vi "simon.vi"() -> ()   [LabVIEW 2024]
uses:
  state machine controller.ctl
  VI Communication.ctl
  HTTP_helpers/session.vi
  HTTP_helpers/user_name.vi
panel:
  in  "UI Controller":T1(tab)
  in  "Home page open leaderboard":bool caption="open leaderboard"
  in  "Home page login button":bool
  in  "Home page check rules":bool caption="Blank Button"
  in  "confirm login":bool
  in  "Login page go back":bool caption="Blank Button"
  in  "Login Password":string
  in  "User Name":string
  in  "Afterlogin Logout Button":bool
  out "user highest score achieved time":string
  out "user highest score":string
  out "Avatar":picture
  out "Afterlogin show user name":string
  in  "Afterlogin check leaderboard":bool caption="open leaderboard"
  in  "Afterlogin play":bool
  in  "AfterLogin home check rules":bool caption="Blank Button"
  in  "New Game":bool
  in  "Local Save":bool
  in  "Cloud Save":bool
  in  "How to start go back":bool caption="Blank Button"
  in  "Play Game":bool caption="Blank Button"
  in  "Difficulty":dbl(slide) scale=1.0..10.0
  in  "Difficulty go back":bool caption="Blank Button"
  in  "Game page EXIT":bool caption="Blank Button"
  out "Save Path":path
  out "Level":dbl
  out "Score":dbl
  in  "Pause Game Back to Home":bool
  # "Size 481 * 730"
  # "Simon Game"
  # "Login to play"
  # "Login or Register"
  # "User Name"
  # "Password"
  # "If you don't have an account yet, we will create one for you"
  # "Welcome"
  # "Simon Game"
  # "My highest score:"
  # "Achieved at:"
  # "How do you wanna start?"
  # "Your game will be automatically saved to server and \n./data/saves for local while playing"
  # "Difficulty?"
  # "Recommended"
  # "↓"
  # "Eazzzzzy"
  # "Hard"
  # "Your choice of difficulty will be counted in the score calculation"
  # "Session Finished"
  # "Score"
  # "Level"
  # "Save Path"
  # "Your game process is already saved on server"
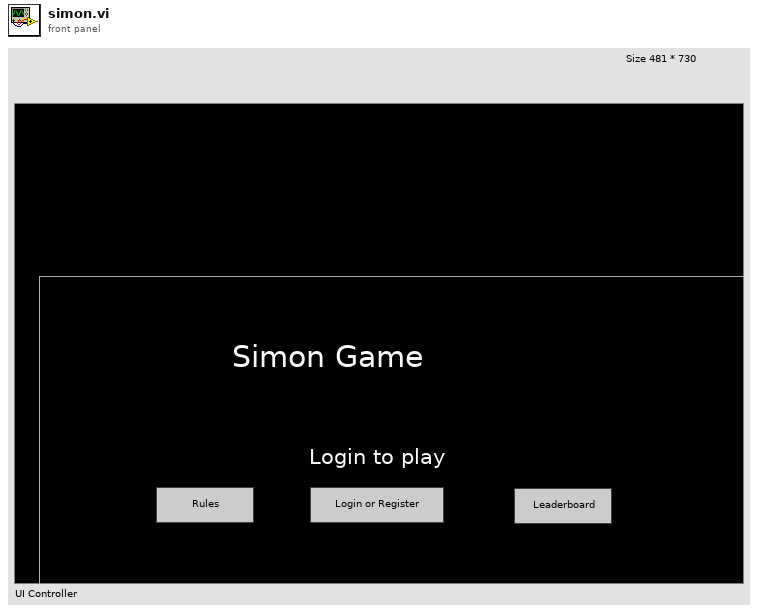
[diagram p1: front panel]
types:
  T1 = enum32{"Home Page", "Login Page", "AfterLogin Home", "How to Start", "New Game Difficulty", "Game Page", "Pause Game"}
  T2 = typedef "state machine controller.ctl" = cluster{"State Machine State":string, "Difficulty":dbl, "Login User Name":string, "Login User Passwd":string}
  T3 = enum32{"Home Page", "Login Page", "AfterLogin Home", "How to Start", "New Game Difficulty", "Game Page"}
  T4 = enum8{"Enabled", "Disabled", "Disabled and Grayed Out"}
  T5 = typedef "LVRectTypeDef.ctl" = cluster{"Left":i16, "Top":i16, "Right":i16, "Bottom":i16}
  T6 = typedef "imagedata.ctl" = cluster{"image type":i32, "image depth":i32, "image":u8[], "mask":u8[], "colors":u32[], "Rectangle":cluster{"left":i16, "top":i16, "right":i16, "bottom":i16}}
  T7 = typedef "VI Communication.ctl" = cluster{"Queue":refnum<queue>, "Path":path, "Score":dbl, "Level":dbl}
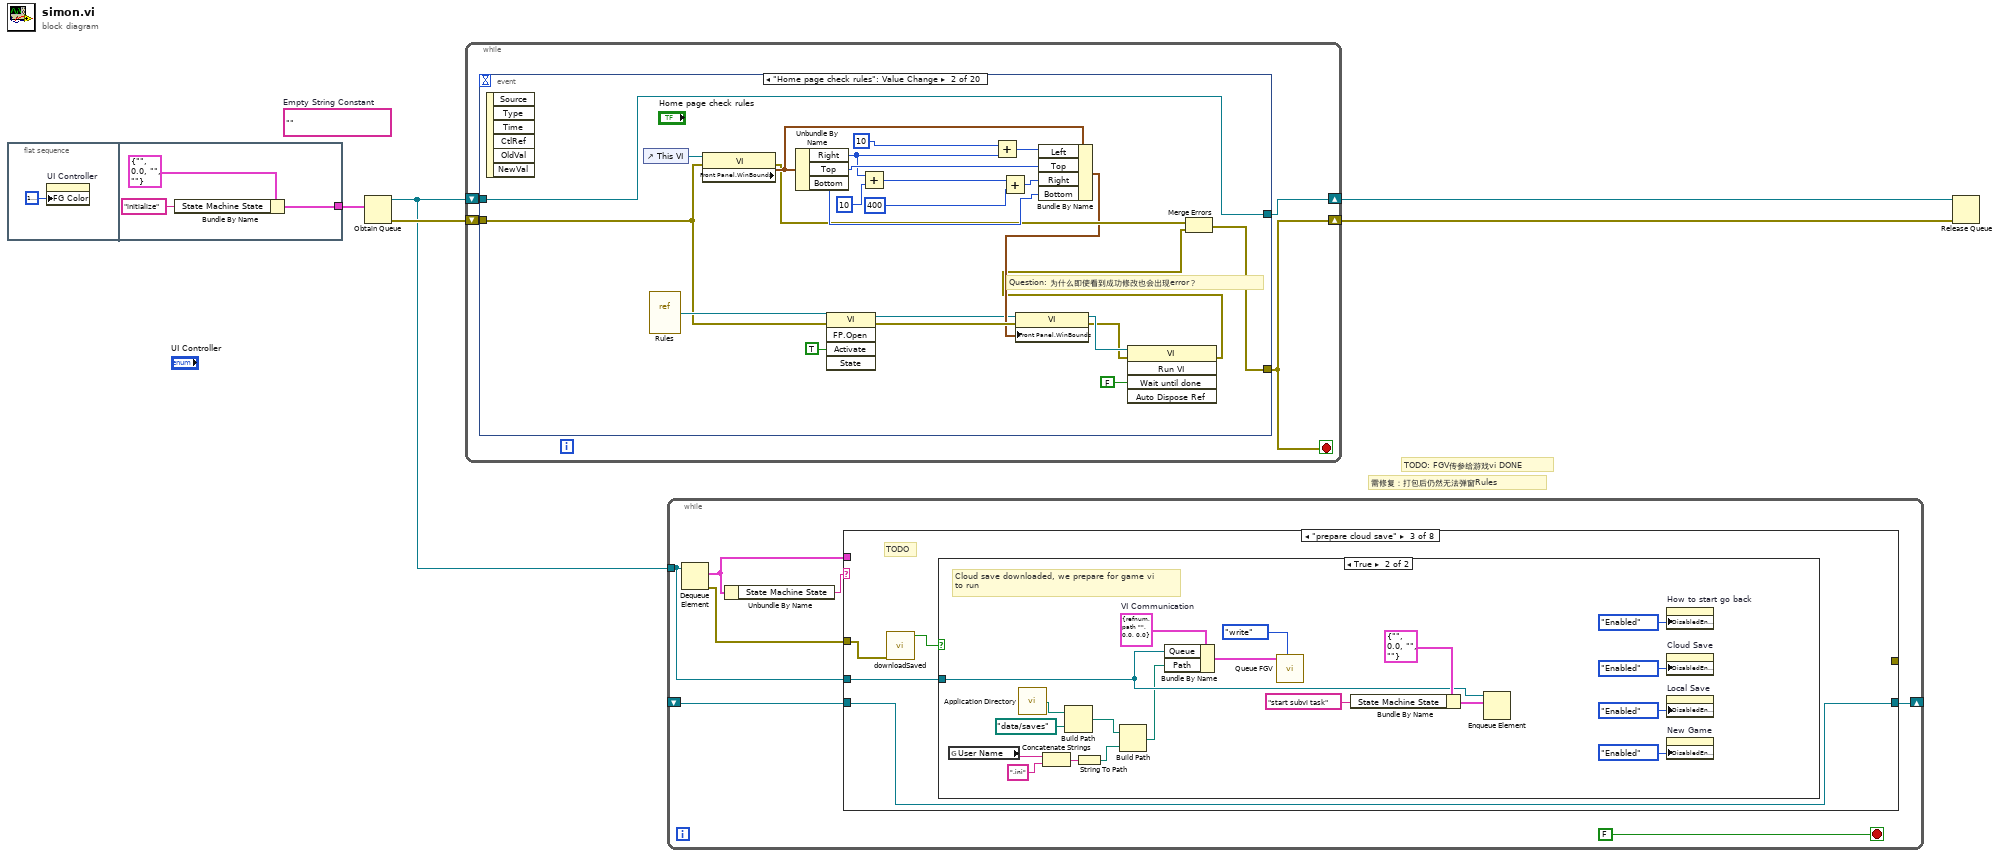
[diagram p0: block diagram]
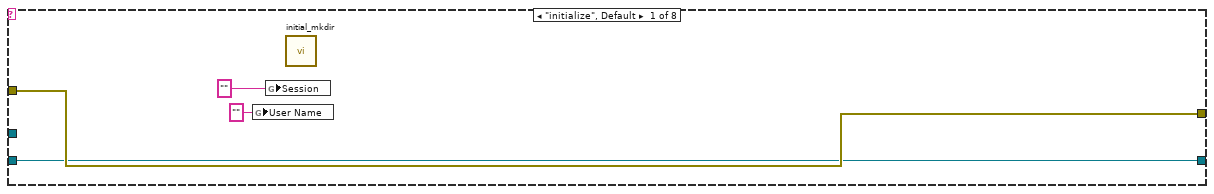
[diagram p2: hidden frame]
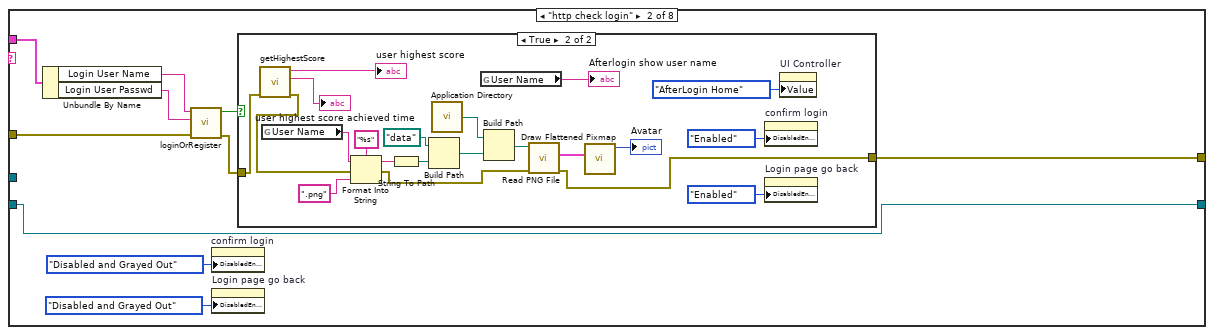
[diagram p3: hidden frame]
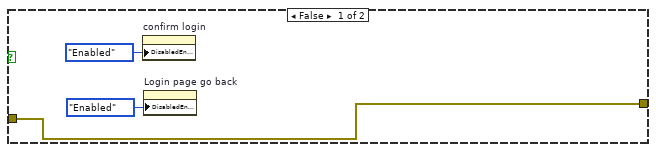
[diagram p4: hidden frame]
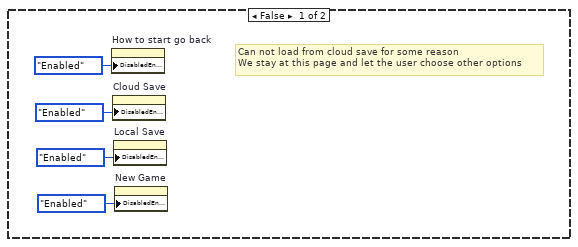
[diagram p5: hidden frame]
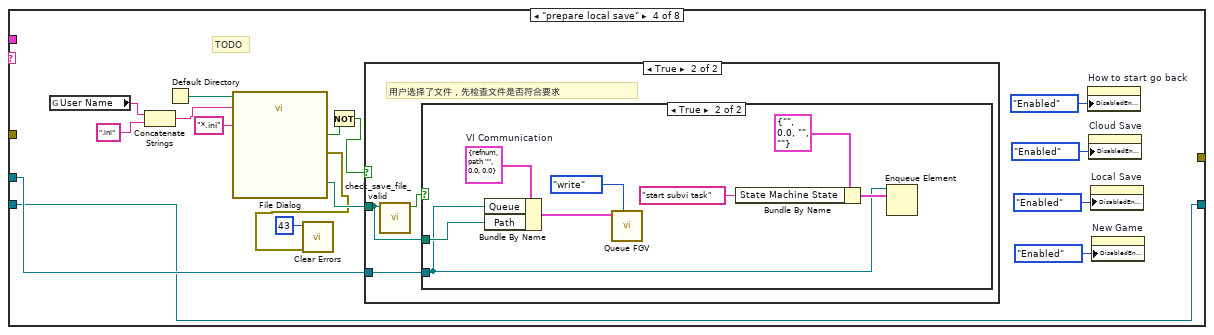
[diagram p6: hidden frame]
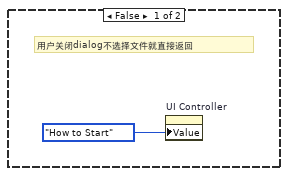
[diagram p7: hidden frame]
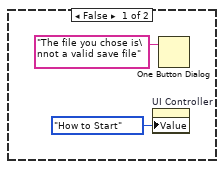
[diagram p8: hidden frame]
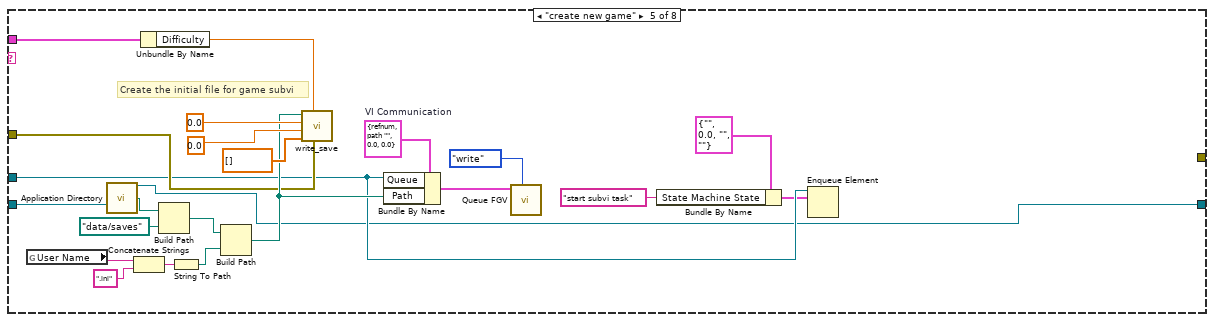
[diagram p9: hidden frame]
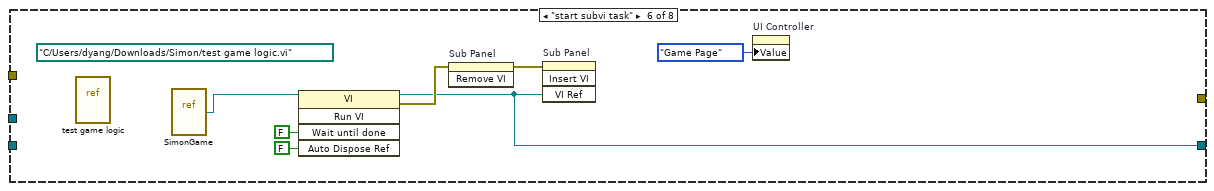
[diagram p10: hidden frame]
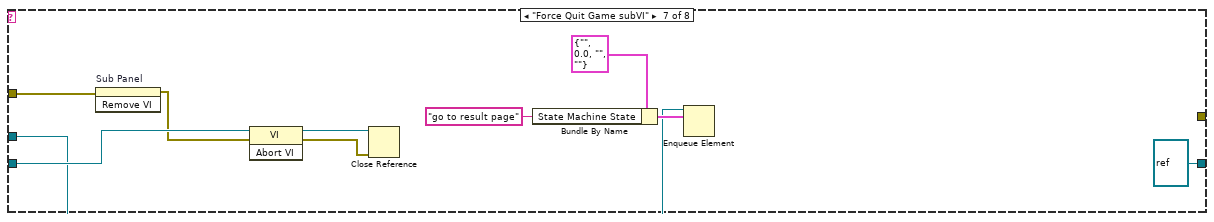
[diagram p11: hidden frame]
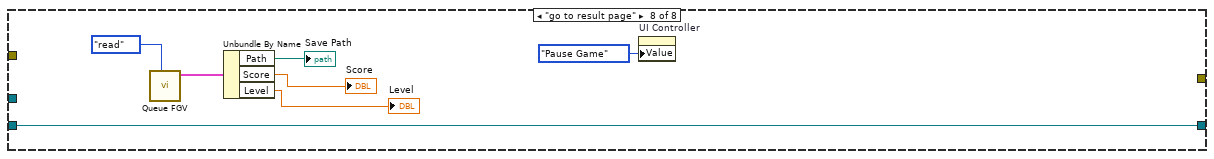
[diagram p12: hidden frame]
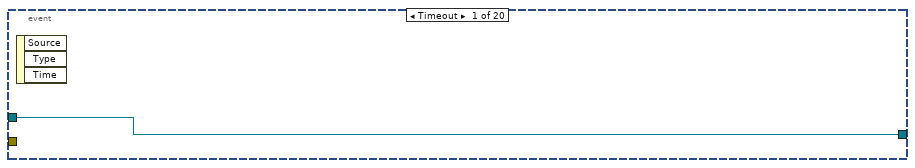
[diagram p13: hidden frame]
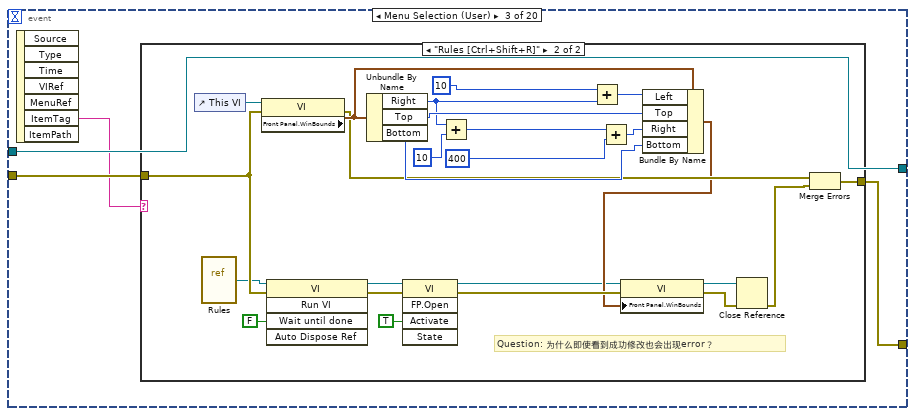
[diagram p14: hidden frame]
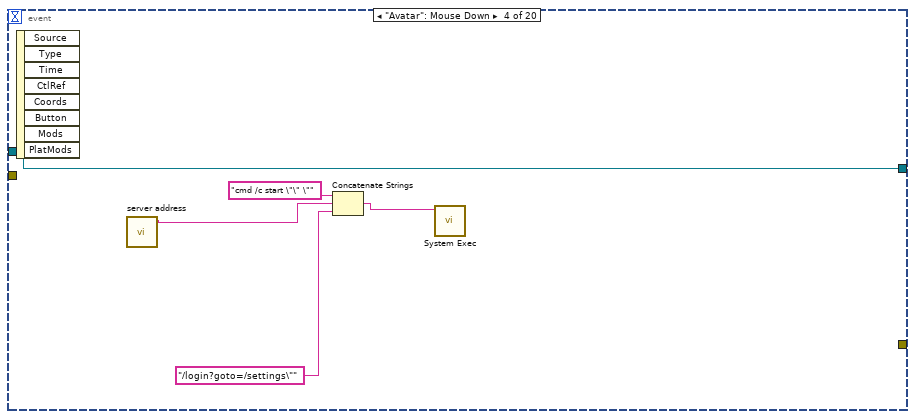
[diagram p16: hidden frame]
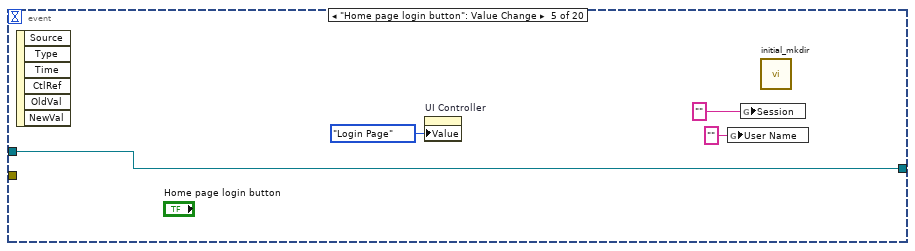
[diagram p17: hidden frame]
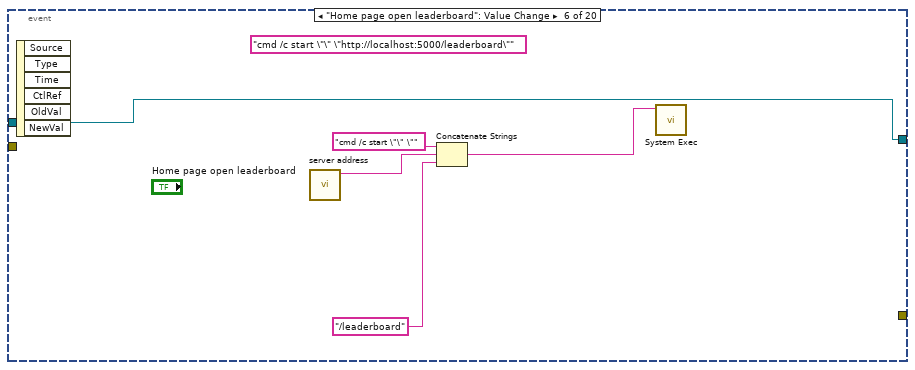
[diagram p18: hidden frame]
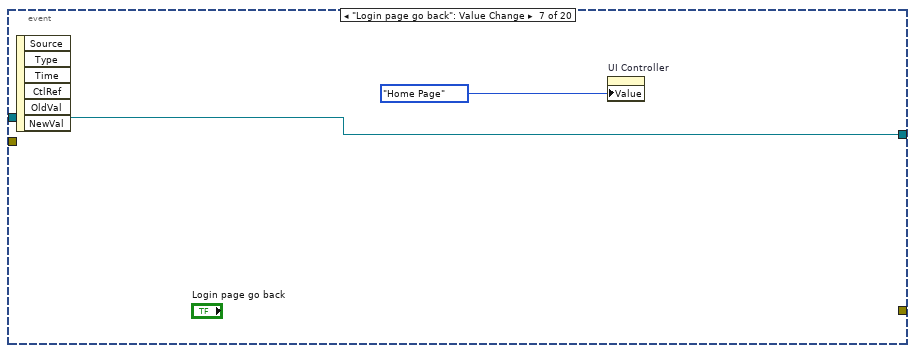
[diagram p19: hidden frame]
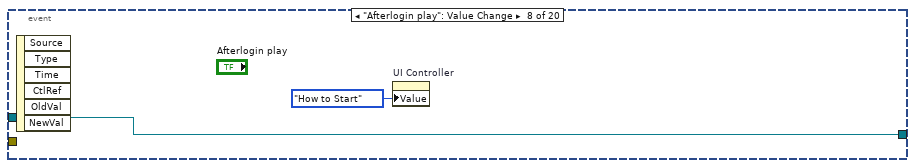
[diagram p20: hidden frame]
diagram:
  (unwired) ""  # Empty String Constant
  # "需修复：打包后仍然无法弹窗Rules"
  # "TODO: FGV传参给游戏vi DONE"
  n1 = flat-sequence {
    tunnel: [w7] -> w1
    frame #0 {
      n2 = property on="UI Controller" class="TabCtl (strict)"("FG Color"=u32 16777222 ("Colors:BG Color")) -> ()  [unwired: 2 in, 2 out]
    }
    frame #1 {
      n3 = Bundle By Name(cluster=T2 {"State Machine State"="", "Difficulty"=0.0, "Login User Name"="", "Login User Passwd"=""} ("Cluster"), "State Machine State"="initialize") -> (w7:T2)
    }
  }
  n4 = Obtain Queue(element data type=w1) -> (queue out=w2:refnum<queue>, error out=w5:errorcluster)  [unwired: 4 in, 1 out]
  n5 = while {
    shift-right: [w12] -> w4
    shift-left: w5 -> [w13]
    shift-right: [w11] -> w3
    shift-left: w2 -> [w10]
    stop <- w12 stop-if-true
    n6 = event shown="[1] \"Home page check rules\": Value Change" {
      selector: _ -> [_ _ _ _ _ _ _ _ _ _ _ _ _ _ _ _ _ _ _ _]
      dyn-events: _ -> [_ _ _ _ _ _ _ _ _ _ _ _ _ _ _ _ _ _ _ _]
      timeout: _ -> [_ _ _ _ _ _ _ _ _ _ _ _ _ _ _ _ _ _ _ _]
      tunnel: w13 -> [_ w18 w41 _ _ _ _ _ _ _ _ _ _ _ _ _ _ w134 _ _]
      tunnel: w10 -> [w14 w26 w42 w73 w76 w78 w83 w86 w88 w97 w106 w108 w110 w112 w118 w125 w127 w133 w161 w166]
      tunnel: [_ w25 w40 _ _ _ _ _ _ _ _ _ _ _ _ _ _ w138 _ _] -> w12
      tunnel: [w14 w26 w42 w73 w76 w78 w83 w86 w88 w96 w105 w108 w110 w113 w117 w125 w126 w133 w161 w166] -> w11
      event Timeout {
        n7 = event-data() -> ()  [unwired: 1 in, 3 out]
      }
      event "Home page check rules": Value Change {
        # "Question: 为什么即使看到成功修改也会出现error？"
        n8 = event-data() -> ()  [unwired: 1 in, 6 out]
        n9 = control-ref of="This VI"() -> (w38:refnum<vi>)
        n10 = vi-ref "Rules.vi"() -> (w19:refnum<vi>)
        n11 = property class="VI"(reference=w38, error in=w18) -> (error out=w27:errorcluster, "Front Panel.WinBounds"=w36:T5)  [unwired: 1 out]
        n12 = Unbundle By Name(w36) -> ("Right"=w33:i16, "Top"=w34:i16, "Bottom"=w28:i16)
        n13 = invoke class="VI" method="FP.Open"(reference=w19, error in=w18, "Activate"=TRUE ("Activate?")) -> (reference out=w20:refnum<vi>, error out=w22:errorcluster)  [unwired: 2 in, 3 out]
        n14 = Add(x=w33, y=i16 10) -> (x+y=w31:i16)
        n15 = Add(x=i16 10, y=w33) -> (x+y=w35:i16)
        n16 = Add(x=w31, y=i16 400) -> (x+y=w29:i16)
        n17 = Bundle By Name(cluster=w36, "Left"=w35, "Top"=w34, "Right"=w29, "Bottom"=w28) -> (w21:T5)
        n18 = property class="VI"(reference=w20, error in=w22, "Front Panel.WinBounds"=w21) -> (reference out=w17:refnum<vi>, error out=w16:errorcluster)
        n19 = invoke class="VI" method="Run VI"(reference=w17, error in=w16, "Wait until done"=FALSE ("Wait Until Done")) -> (error out=w15:errorcluster)  [unwired: 2 in, 4 out]
        n20 = Merge Errors(w27, w15) -> (w25:errorcluster)
      }
      event Menu Selection (User) {
        n21 = event-data() -> ("ItemTag"=w39:string)  [unwired: 1 in, 6 out]
        n22 = case shown="\"Rules [Ctrl+Shift+R]\"" w39 {
          tunnel: w41 -> [w43 w56]
          tunnel: [w43 w55] -> w40
          frame Default {
          }
          frame "Rules [Ctrl+Shift+R]" {
            # "Question: 为什么即使看到成功修改也会出现error？"
            n23 = control-ref of="This VI"() -> (w68:refnum<vi>)
            n24 = vi-ref "Rules.vi"() -> (w47:refnum<vi>)
            n25 = property class="VI"(reference=w68, error in=w56) -> (error out=w57:errorcluster, "Front Panel.WinBounds"=w66:T5)  [unwired: 1 out]
            n26 = invoke class="VI" method="Run VI"(reference=w47, error in=w56, "Wait until done"=FALSE ("Wait Until Done")) -> (reference out=w52:refnum<vi>, error out=w50:errorcluster)  [unwired: 2 in, 3 out]
            n27 = Unbundle By Name(w66) -> ("Right"=w63:i16, "Top"=w64:i16, "Bottom"=w58:i16)
            n28 = invoke class="VI" method="FP.Open"(reference=w52, error in=w50, "Activate"=TRUE ("Activate?")) -> (reference out=w44:refnum<vi>, error out=w46:errorcluster)  [unwired: 2 in, 3 out]
            n29 = Add(x=w63, y=i16 10) -> (x+y=w61:i16)
            n30 = Add(x=i16 10, y=w63) -> (x+y=w65:i16)
            n31 = Add(x=w61, y=i16 400) -> (x+y=w59:i16)
            n32 = Bundle By Name(cluster=w66, "Left"=w65, "Top"=w64, "Right"=w59, "Bottom"=w58) -> (w45:T5)
            n33 = property class="VI"(reference=w44, error in=w46, "Front Panel.WinBounds"=w45) -> (reference out=w49:refnum<vi>, error out=w48:errorcluster)
            n34 = Close Reference(reference=w49, error in (no error)=w48) -> (error out=w54:errorcluster)
            n35 = Merge Errors(w57, w54) -> (w55:errorcluster)
          }
        }
      }
      event "Avatar": Mouse Down {
        n36 = event-data() -> ()  [unwired: 1 in, 8 out]
        n37 = call "server address.vi"() -> ("Server Address"=w70:string)  [unwired: 11 in]
        n38 = Concatenate Strings("cmd /c start \"\" \"" ("string"), w70, "/login?goto=/settings\"" ("string")) -> (w69:string)
        n39 = call <vilib>:"System Exec.vi"("command line"=w69) -> ()  [unwired: 7 in, 4 out]
      }
      event "Home page login button": Value Change {
        n40 = event-data() -> ()  [unwired: 1 in, 6 out]
        n41 = property on="UI Controller" class="TabCtl (strict)"("Value"=T3."Login Page" ("UI Controller")) -> ()  [unwired: 2 in, 2 out]
        n42 = global write "user_name.vi" "User Name"("" ("User Name")) -> ()
        n43 = global write "session.vi" "Session"("" ("Session")) -> ()
        n44 = call "initial_mkdir.vi"() -> ()  [unwired: 11 in, 1 out]
      }
      event "Home page open leaderboard": Value Change {
        (unwired) "cmd /c start \"\" \"http://localhost:5000/leaderboard\"" ("command line")
        n45 = event-data() -> ()  [unwired: 1 in, 6 out]
        n46 = call "server address.vi"() -> ("Server Address"=w81:string)  [unwired: 11 in]
        n47 = Concatenate Strings("cmd /c start \"\" \"" ("string"), w81, "/leaderboard" ("string")) -> (w79:string)
        n48 = call <vilib>:"System Exec.vi"("command line"=w79) -> ()  [unwired: 7 in, 4 out]
      }
      event "Login page go back": Value Change {
        n49 = event-data() -> ()  [unwired: 1 in, 6 out]
        n50 = property on="UI Controller" class="TabCtl (strict)"("Value"=T3."Home Page" ("UI Controller")) -> ()  [unwired: 2 in, 2 out]
      }
      event "Afterlogin play": Value Change {
        n51 = event-data() -> ()  [unwired: 1 in, 6 out]
        n52 = property on="UI Controller" class="TabCtl (strict)"("Value"=T3."How to Start" ("UI Controller")) -> ()  [unwired: 2 in, 2 out]
      }
      event "How to start go back": Value Change {
        n53 = event-data() -> ()  [unwired: 1 in, 6 out]
        n54 = property on="UI Controller" class="TabCtl (strict)"("Value"=T3."AfterLogin Home" ("UI Controller")) -> ()  [unwired: 2 in, 2 out]
      }
      event "Cloud Save": Value Change {
        # "Check & Load Cloud Save from server"
        n55 = event-data() -> ()  [unwired: 1 in, 6 out]
        n56 = property on="Cloud Save" class="Bool"("DisabledEnum"=T4."Disabled and Grayed Out" ("Disabled")) -> ()  [unwired: 2 in, 2 out]
        n57 = property on="Local Save" class="Bool"("DisabledEnum"=T4."Disabled and Grayed Out" ("Disabled")) -> ()  [unwired: 2 in, 2 out]
        n58 = property on="How to start go back" class="Bool"("DisabledEnum"=T4."Disabled and Grayed Out" ("Disabled")) -> ()  [unwired: 2 in, 2 out]
        n59 = Bundle By Name(cluster=T2 {"State Machine State"="", "Difficulty"=0.0, "Login User Name"="", "Login User Passwd"=""} ("Cluster"), "State Machine State"="prepare cloud save") -> (w93:T2)
        n60 = Enqueue Element(queue=w97, element=w93) -> (queue out=w96:refnum<queue>)  [unwired: 2 in, 2 out]
        n61 = property on="New Game" class="Bool"("DisabledEnum"=T4."Disabled and Grayed Out" ("Disabled")) -> ()  [unwired: 2 in, 2 out]
      }
      event "Local Save": Value Change {
        n62 = event-data() -> ()  [unwired: 1 in, 6 out]
        n63 = property on="How to start go back" class="Bool"("DisabledEnum"=T4."Disabled and Grayed Out" ("Disabled")) -> ()  [unwired: 2 in, 2 out]
        n64 = property on="Cloud Save" class="Bool"("DisabledEnum"=T4."Disabled and Grayed Out" ("Disabled")) -> ()  [unwired: 2 in, 2 out]
        n65 = property on="Local Save" class="Bool"("DisabledEnum"=T4."Disabled and Grayed Out" ("Disabled")) -> ()  [unwired: 2 in, 2 out]
        n66 = property on="New Game" class="Bool"("DisabledEnum"=T4."Disabled and Grayed Out" ("Disabled")) -> ()  [unwired: 2 in, 2 out]
        n67 = Bundle By Name(cluster=T2 {"State Machine State"="", "Difficulty"=0.0, "Login User Name"="", "Login User Passwd"=""} ("Cluster"), "State Machine State"="prepare local save") -> (w102:T2)
        n68 = Enqueue Element(queue=w106, element=w102) -> (queue out=w105:refnum<queue>)  [unwired: 2 in, 2 out]
      }
      event "New Game": Value Change {
        n69 = event-data() -> ()  [unwired: 1 in, 6 out]
        n70 = property on="UI Controller" class="TabCtl (strict)"("Value"=T3."New Game Difficulty" ("UI Controller")) -> ()  [unwired: 2 in, 2 out]
      }
      event "Difficulty go back": Value Change {
        n71 = event-data() -> ()  [unwired: 1 in, 6 out]
        n72 = property on="UI Controller" class="TabCtl (strict)"("Value"=T3."How to Start" ("UI Controller")) -> ()  [unwired: 2 in, 2 out]
      }
      event "Play Game": Value Change {
        n73 = event-data() -> ()  [unwired: 1 in, 6 out]
        n74 = Bundle By Name(cluster=T2 {"State Machine State"="", "Difficulty"=0.0, "Login User Name"="", "Login User Passwd"=""} ("Cluster"), "State Machine State"="create new game", "Difficulty"="Difficulty") -> (w111:T2)
        n75 = Enqueue Element(queue=w112, element=w111) -> (queue out=w113:refnum<queue>)  [unwired: 2 in, 2 out]
      }
      event "Game page EXIT": Value Change {
        n76 = event-data() -> ()  [unwired: 1 in, 6 out]
        n77 = Bundle By Name(cluster=T2 {"State Machine State"="", "Difficulty"=0.0, "Login User Name"="", "Login User Passwd"=""} ("Cluster"), "State Machine State"="Force Quit Game subVI") -> (w119:T2)
        n78 = Enqueue Element(queue=w118, element=w119) -> (queue out=w117:refnum<queue>)  [unwired: 2 in, 2 out]
      }
      event "Pause Game Back to Home": Value Change {
        n79 = event-data() -> ()  [unwired: 1 in, 6 out]
        n80 = call "getHighestScore.vi"() -> ("Highest Score Achineved Time"=w122:string, "Highest Score"=w123:string)  [unwired: 9 in, 1 out]
        n81 = property on="user highest score" class="Str"("Value"=w123) -> ()  [unwired: 2 in, 2 out]
        n82 = property on="user highest score achieved time" class="Str"("Value"=w122) -> ()  [unwired: 2 in, 2 out]
        n83 = property on="UI Controller" class="TabCtl (strict)"("Value"=T1."AfterLogin Home" ("UI Controller")) -> ()  [unwired: 2 in, 2 out]
      }
      event "confirm login": Value Change {
        n84 = event-data() -> ()  [unwired: 1 in, 6 out]
        n85 = Bundle By Name(cluster=T2 {"State Machine State"="", "Difficulty"=0.0, "Login User Name"="", "Login User Passwd"=""} ("Cluster"), "State Machine State"="http check login", "Login User Name"="User Name", "Login User Passwd"="Login Password") -> (w128:T2)
        n86 = Enqueue Element(queue=w127, element=w128) -> (queue out=w126:refnum<queue>)  [unwired: 2 in, 2 out]
      }
      event "AfterLogin home check rules": Value Change {
        # "Question: 为什么即使看到成功修改也会出现error？"
        n87 = event-data() -> ()  [unwired: 1 in, 6 out]
        n88 = control-ref of="This VI"() -> (w152:refnum<vi>)
        n89 = Open VI Reference(vi path=path "C:/Users/dyang/Downloads/Simon/Rules.vi", error in (no error)=w134) -> (vi reference=w155:refnum<vi>, error out=w160:errorcluster)  [unwired: 4 in]
        n90 = property class="VI"(reference=w152, error in=w134) -> (error out=w135:errorcluster, "Front Panel.WinBounds"=w150:T5)  [unwired: 1 out]
        n91 = invoke class="VI" method="Run VI"(reference=w155, error in=w160, "Wait until done"=FALSE ("Wait Until Done")) -> (reference out=w158:refnum<vi>, error out=w156:errorcluster)  [unwired: 2 in, 3 out]
        n92 = Unbundle By Name(w150) -> ("Right"=w146:i16, "Top"=w148:i16, "Bottom"=w141:i16)
        n93 = invoke class="VI" method="FP.Open"(reference=w158, error in=w156, "Activate"=TRUE ("Activate?")) -> (reference out=w154:refnum<vi>, error out=w153:errorcluster)  [unwired: 2 in, 3 out]
        n94 = Add(x=w146, y=i16 10) -> (x+y=w144:i16)
        n95 = Add(x=i16 10, y=w146) -> (x+y=w149:i16)
        n96 = Add(x=w144, y=i16 400) -> (x+y=w142:i16)
        n97 = Bundle By Name(cluster=w150, "Left"=w149, "Top"=w148, "Right"=w142, "Bottom"=w141) -> (w147:T5)
        n98 = property class="VI"(reference=w154, error in=w153, "Front Panel.WinBounds"=w147) -> (error out=w136:errorcluster)  [unwired: 1 out]
        n99 = Merge Errors(w135, w136) -> (w137:errorcluster)
        n100 = call <vilib>:"Clear Errors.vi"("error in (no error)"=w137, "specific error code to clear (0: all)"=1) -> ("error out"=w138:errorcluster)  [unwired: 4 in, 1 out]
      }
      event "Afterlogin check leaderboard": Value Change {
        n101 = event-data() -> ()  [unwired: 1 in, 6 out]
        n102 = call "server address.vi"() -> ("Server Address"=w164:string)  [unwired: 11 in]
        n103 = Concatenate Strings("cmd /c start \"\" \"" ("string"), w164, "/leaderboard" ("string")) -> (w162:string)
        n104 = call <vilib>:"System Exec.vi"("command line"=w162) -> ()  [unwired: 7 in, 4 out]
      }
      event "Afterlogin Logout Button": Value Change {
        n105 = event-data() -> ()  [unwired: 1 in, 6 out]
        n106 = property on="UI Controller" class="TabCtl (strict)"("Value"=T3."Home Page" ("UI Controller")) -> ()  [unwired: 2 in, 2 out]
        n107 = global write "user_name.vi" "User Name"("" ("User Name")) -> ()
        n108 = global write "session.vi" "Session"("" ("Session")) -> ()
      }
    }
  }
  n109 = while {
    tunnel: w2 -> [w172]
    shift-right: [w171] -> _
    shift-left: _ -> [w170]
    stop <- FALSE stop-if-true
    n110 = Dequeue Element(queue=w172) -> (element=w175:T2, error out=w174:errorcluster)  [unwired: 2 in, 2 out]
    n111 = Unbundle By Name(w175) -> ("State Machine State"=w173:string)
    n112 = case shown="\"prepare cloud save\"" w173 {
      tunnel: w175 -> [_ w190 _ _ w290 _ _ _]
      tunnel: w174 -> [w178 w183 w218 _ w277 _ w310 _]
      tunnel: [w178 w182 _ _ _ _ _ _] -> _
      tunnel: w172 -> [_ _ w216 w247 w276 _ w301 _]
      tunnel: [w177 w181 w215 w246 w272 w296 refnum<vi> refnum ("vi reference") w317] -> w171
      tunnel: w170 -> [w177 w181 w215 w246 w272 _ w309 w317]
      frame "initialize", Default {
        n113 = global write "user_name.vi" "User Name"("" ("User Name")) -> ()
        n114 = global write "session.vi" "Session"("" ("Session")) -> ()
        n115 = call "initial_mkdir.vi"() -> ()  [unwired: 11 in, 1 out]
      }
      frame "http check login" {
        n116 = Unbundle By Name(w190) -> ("Login User Name"=w189:string, "Login User Passwd"=w188:string)
        n117 = call "loginOrRegister.vi"("error in"=w183, "passwd"=w188, "uname"=w189) -> ("error out"=w184:errorcluster, "OK?"=w187:bool)  [unwired: 7 in]
        n118 = property on="confirm login" class="Bool"("DisabledEnum"=T4."Disabled and Grayed Out" ("Disabled")) -> ()  [unwired: 2 in, 2 out]
        n119 = property on="Login page go back" class="Bool"("DisabledEnum"=T4."Disabled and Grayed Out" ("Disabled")) -> ()  [unwired: 2 in, 2 out]
        n120 = case shown="True" w187 {
          tunnel: w184 -> [w191 w196]
          tunnel: [w191 w194] -> w182
          frame False {
            n121 = property on="confirm login" class="Bool"("DisabledEnum"=T4."Enabled" ("Disabled")) -> ()  [unwired: 2 in, 2 out]
            n122 = property on="Login page go back" class="Bool"("DisabledEnum"=T4."Enabled" ("Disabled")) -> ()  [unwired: 2 in, 2 out]
          }
          frame True {
            n123 = call "getHighestScore.vi"("error in"=w196) -> ("error out"=w195:errorcluster, "Highest Score Achineved Time"=→"user highest score achieved time":string, "Highest Score"=→"user highest score":string)  [unwired: 8 in]
            n124 = global read "user_name.vi" "User Name"() -> (w207:string)
            n125 = Format Into String(format string="%s", initial string=w207, error in=w195, ".png" ("input 1")) -> (resulting string=w206:string, error out=w197:errorcluster)
            n126 = String To Path(string=w206) -> (path=w205:path)
            n127 = Build Path(base path=path "data", name or relative path=w205) -> (appended path=w203:path)
            n128 = call <vilib>:"Application Directory.vi"() -> ("Application Directory"=w202:path)
            n129 = global read "user_name.vi" "User Name"() -> (→"Afterlogin show user name":string)
            n130 = Build Path(base path=w202, name or relative path=w203) -> (appended path=w201:path)
            n131 = call <vilib>:"Read PNG File.vi"("error in (no error)"=w197, "path to PNG file"=w201) -> ("error out"=w194:errorcluster, "image data"=w200:T6)  [unwired: 7 in, 1 out]
            n132 = call <vilib>:"Draw Flattened Pixmap.vi"("image data"=w200) -> ("new picture"=→"Avatar":picture)  [unwired: 8 in]
            n133 = property on="confirm login" class="Bool"("DisabledEnum"=T4."Enabled" ("Disabled")) -> ()  [unwired: 2 in, 2 out]
            n134 = property on="Login page go back" class="Bool"("DisabledEnum"=T4."Enabled" ("Disabled")) -> ()  [unwired: 2 in, 2 out]
            n135 = property on="UI Controller" class="TabCtl (strict)"("Value"=T3."AfterLogin Home" ("UI Controller")) -> ()  [unwired: 2 in, 2 out]
          }
        }
      }
      frame "prepare cloud save" {
        # "TODO"
        n136 = call "downloadSaved.vi"("error in"=w218) -> ("OK?"=w217:bool)  [unwired: 9 in, 1 out]
        n137 = case shown="True" w217 {
          tunnel: w216 -> [_ w224]
          frame False {
            # "Can not load from cloud save for some reason\nWe stay at this page and let the user choose other options"
            n138 = property on="How to start go back" class="Bool"("DisabledEnum"=T4."Enabled" ("Disabled")) -> ()  [unwired: 2 in, 2 out]
            n139 = property on="Cloud Save" class="Bool"("DisabledEnum"=T4."Enabled" ("Disabled")) -> ()  [unwired: 2 in, 2 out]
            n140 = property on="Local Save" class="Bool"("DisabledEnum"=T4."Enabled" ("Disabled")) -> ()  [unwired: 2 in, 2 out]
            n141 = property on="New Game" class="Bool"("DisabledEnum"=T4."Enabled" ("Disabled")) -> ()  [unwired: 2 in, 2 out]
          }
          frame True {
            w229 = T7 {"Queue"=refnum, "Path"=path "", "Score"=0.0, "Level"=0.0}  # VI Communication
            # "Cloud save downloaded, we prepare for game vi\nto run"
            n142 = global read "user_name.vi" "User Name"() -> (w233:string)
            n143 = call <vilib>:"Application Directory.vi"() -> ("Application Directory"=w237:path)
            n144 = Concatenate Strings(w233, ".ini" ("string")) -> (w235:string)
            n145 = Build Path(base path=w237, name or relative path=path "data/saves") -> (appended path=w232:path)
            n146 = String To Path(string=w235) -> (path=w231:path)
            n147 = Build Path(base path=w232, name or relative path=w231) -> (appended path=w223:path)
            n148 = Bundle By Name(cluster=w229, "Queue"=w224, "Path"=w223) -> (w228:T7)
            n149 = call "Queue FGV.vi"("Enum"=enum16{"read", "write"}."write", "VI Communication In"=w228) -> ()  [unwired: 9 in, 1 out]
            n150 = Bundle By Name(cluster=T2 {"State Machine State"="", "Difficulty"=0.0, "Login User Name"="", "Login User Passwd"=""} ("Cluster"), "State Machine State"="start subvi task") -> (w226:T2)
            n151 = Enqueue Element(queue=w224, element=w226) -> ()  [unwired: 2 in, 3 out]
            n152 = property on="How to start go back" class="Bool"("DisabledEnum"=T4."Enabled" ("Disabled")) -> ()  [unwired: 2 in, 2 out]
            n153 = property on="Cloud Save" class="Bool"("DisabledEnum"=T4."Enabled" ("Disabled")) -> ()  [unwired: 2 in, 2 out]
            n154 = property on="Local Save" class="Bool"("DisabledEnum"=T4."Enabled" ("Disabled")) -> ()  [unwired: 2 in, 2 out]
            n155 = property on="New Game" class="Bool"("DisabledEnum"=T4."Enabled" ("Disabled")) -> ()  [unwired: 2 in, 2 out]
          }
        }
      }
      frame "prepare local save" {
        # "TODO"
        n156 = global read "user_name.vi" "User Name"() -> (w250:string)
        n157 = Concatenate Strings(w250, ".ini" ("string")) -> (w249:string)
        n158 = Default Directory() -> (w253:path)
        n159 = call "File Dialog"("start path"=w253, "default name"=w249, "pattern (all files)"="*.ini") -> ("selected path"=w248:path, "cancelled"=w245:bool, "error out"=w242:errorcluster)  [unwired: 9 in, 1 out]
        n160 = call <vilib>:"Clear Errors.vi"("error in (no error)"=w242, "specific error code to clear (0: all)"=43) -> ()  [unwired: 4 in, 2 out]
        n161 = Not(x=w245) -> (.not. x?=w244:bool)
        n162 = case shown="True" w244 {
          tunnel: w248 -> [_ w259]
          tunnel: w247 -> [_ w260]
          frame False {
            # "用户关闭dialog不选择文件就直接返回"
            n163 = property on="UI Controller" class="TabCtl (strict)"("Value"=T3."How to Start" ("UI Controller")) -> ()  [unwired: 2 in, 2 out]
          }
          frame True {
            # "用户选择了文件，先检查文件是否符合要求"
            n164 = call "check_save_file_valid.vi"("save file path"=w259) -> ("valid?"=w261:bool)  [unwired: 9 in, 1 out]
            n165 = case shown="True" w261 {
              tunnel: w260 -> [_ w264]
              tunnel: w259 -> [_ w268]
              frame False {
                n166 = property on="UI Controller" class="TabCtl (strict)"("Value"=T3."How to Start" ("UI Controller")) -> ()  [unwired: 2 in, 2 out]
                n167 = One Button Dialog(message="The file you chose is\nnot a valid save file") -> ()  [unwired: 1 in, 1 out]
              }
              frame True {
                w270 = T7 {"Queue"=refnum, "Path"=path "", "Score"=0.0, "Level"=0.0}  # VI Communication
                n168 = Bundle By Name(cluster=w270, "Queue"=w264, "Path"=w268) -> (w269:T7)
                n169 = call "Queue FGV.vi"("Enum"=enum16{"read", "write"}."write", "VI Communication In"=w269) -> ()  [unwired: 9 in, 1 out]
                n170 = Bundle By Name(cluster=T2 {"State Machine State"="", "Difficulty"=0.0, "Login User Name"="", "Login User Passwd"=""} ("Cluster"), "State Machine State"="start subvi task") -> (w266:T2)
                n171 = Enqueue Element(queue=w264, element=w266) -> ()  [unwired: 2 in, 3 out]
              }
            }
          }
        }
        n172 = property on="How to start go back" class="Bool"("DisabledEnum"=T4."Enabled" ("Disabled")) -> ()  [unwired: 2 in, 2 out]
        n173 = property on="Cloud Save" class="Bool"("DisabledEnum"=T4."Enabled" ("Disabled")) -> ()  [unwired: 2 in, 2 out]
        n174 = property on="Local Save" class="Bool"("DisabledEnum"=T4."Enabled" ("Disabled")) -> ()  [unwired: 2 in, 2 out]
        n175 = property on="New Game" class="Bool"("DisabledEnum"=T4."Enabled" ("Disabled")) -> ()  [unwired: 2 in, 2 out]
      }
      frame "create new game" {
        w292 = T7 {"Queue"=refnum, "Path"=path "", "Score"=0.0, "Level"=0.0}  # VI Communication
        # "Create the initial file for game subvi"
        n176 = global read "user_name.vi" "User Name"() -> (w281:string)
        n177 = call <vilib>:"Application Directory.vi"() -> ("Application Directory"=w285:path)
        n178 = Concatenate Strings(w281, ".ini" ("string")) -> (w283:string)
        n179 = Unbundle By Name(w290) -> ("Difficulty"=w289:dbl)
        n180 = Build Path(base path=w285, name or relative path=path "data/saves") -> (appended path=w280:path)
        n181 = String To Path(string=w283) -> (path=w279:path)
        n182 = Build Path(base path=w280, name or relative path=w279) -> (appended path=w278:path)
        n183 = call "write_save.vi"("error in"=w277, "Difficulty"=w289, "Sequence"=dbl[] [], "Level"=0.0, "Score"=0.0, "save file path"=w278) -> ()  [unwired: 5 in, 1 out]
        n184 = Bundle By Name(cluster=w292, "Queue"=w276, "Path"=w278) -> (w291:T7)
        n185 = call "Queue FGV.vi"("Enum"=enum16{"read", "write"}."write", "VI Communication In"=w291) -> ()  [unwired: 9 in, 1 out]
        n186 = Bundle By Name(cluster=T2 {"State Machine State"="", "Difficulty"=0.0, "Login User Name"="", "Login User Passwd"=""} ("Cluster"), "State Machine State"="start subvi task") -> (w274:T2)
        n187 = Enqueue Element(queue=w276, element=w274) -> ()  [unwired: 2 in, 3 out]
      }
      frame "start subvi task" {
        (unwired) path "C:/Users/dyang/Downloads/Simon/test game logic.vi" ("vi path")
        n188 = vi-ref "test game logic.vi"() -> ()  [unwired: 1 out]
        n189 = vi-ref "SimonGame.vi"() -> (w294:refnum<vi>)
        n190 = invoke class="VI" method="Run VI"(reference=w294, "Wait until done"=FALSE ("Wait Until Done"), "Auto Dispose Ref"=FALSE ("Auto Dispose Reference")) -> (reference out=w296:refnum<vi>, error out=w298:errorcluster)  [unwired: 2 in, 3 out]
        n191 = invoke on="Sub Panel" class="SubPnl" method="Remove VI"(error in=w298) -> (error out=w297:errorcluster)  [unwired: 2 in, 2 out]
        n192 = invoke on="Sub Panel" class="SubPnl" method="Insert VI"(error in=w297, "VI Ref"=w296) -> ()  [unwired: 2 in, 4 out]
        n193 = property on="UI Controller" class="TabCtl (strict)"("Value"=T1."Game Page" ("UI Controller")) -> ()  [unwired: 2 in, 2 out]
      }
      frame "Force Quit Game subVI" {
        n194 = invoke on="Sub Panel" class="SubPnl" method="Remove VI"(error in=w310) -> (error out=w305:errorcluster)  [unwired: 2 in, 2 out]
        n195 = invoke class="VI" method="Abort VI"(reference=w309, error in=w305) -> (reference out=w307:refnum<vi>, error out=w306:errorcluster)  [unwired: 1 in, 1 out]
        n196 = Close Reference(reference=w307, error in (no error)=w306) -> ()  [unwired: 1 out]
        n197 = Bundle By Name(cluster=T2 {"State Machine State"="", "Difficulty"=0.0, "Login User Name"="", "Login User Passwd"=""} ("Cluster"), "State Machine State"="go to result page") -> (w303:T2)
        n198 = Enqueue Element(queue=w301, element=w303) -> ()  [unwired: 2 in, 3 out]
      }
      frame "go to result page" {
        n199 = call "Queue FGV.vi"("Enum"=enum16{"read", "write"}."read") -> ("VI Communication Out"=w315:T7)  [unwired: 10 in]
        n200 = Unbundle By Name(w315) -> ("Path"=→"Save Path":path, "Score"=→"Score":dbl, "Level"=→"Level":dbl)
        n201 = property on="UI Controller" class="TabCtl (strict)"("Value"=T1."Pause Game" ("UI Controller")) -> ()  [unwired: 2 in, 2 out]
      }
    }
  }
  n202 = Release Queue(queue=w3, error in (no error)=w4) -> ()  [unwired: 1 in, 3 out]
